vi "Add_Pitot_Vel.vi"(1 "Channels from Client In":string[][](array[string])=[["Data Base:Measurement:Type", "LDA & Cw"], ["Data Base:Position:No of Inst", "2"], ["Data Base:Position:X1", "-60"], ["Data Base:Position:X2", ""], ["Data Base:Position:Y1", "2"], ["Data Base:Position:Y2", "0.00"], ["Data Base:Position:Z1", "0.00"], ["Data Base:Position:Z2", "2.00"]]) -> (0 "Channels from Client Out":string[][](array[string])=[["Data Base:Measurement:Type", "LDA & Cw"], ["Data Base:Position:No of Inst", "2"], ["Data Base:Position:X1", "-60"], ["Data Base:Position:X2", ""], ["Data Base:Position:Y1", "2"], ["Data Base:Position:Y2", "0.00"], ["Data Base:Position:Z1", "0.00"], ["Data Base:Position:Z2", "2.00"]])   [LabVIEW 2011]
uses:
  ADAM Client/Sub VIs/ADAM Controls/Update_scan_value.ctl
  Globals/Meas_global.vi
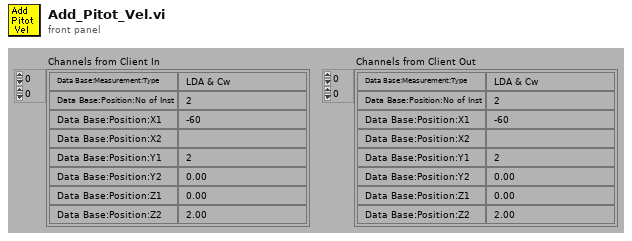
[diagram p1: front panel]
types:
  T1 = typedef "Update_scan_value.ctl" = cluster{"Channel Name":string, "New Value":dbl}
  T2 = typedef "Velocity_cluster.ctl" = cluster{"Name":string, "U":dbl, "u^2":dbl, "u^3/(u^2)^(1.5)":dbl, "u^4/(u^2)^2 -3":dbl, "% u'/U":dbl, "Mean % Err":dbl, "u^4":dbl}
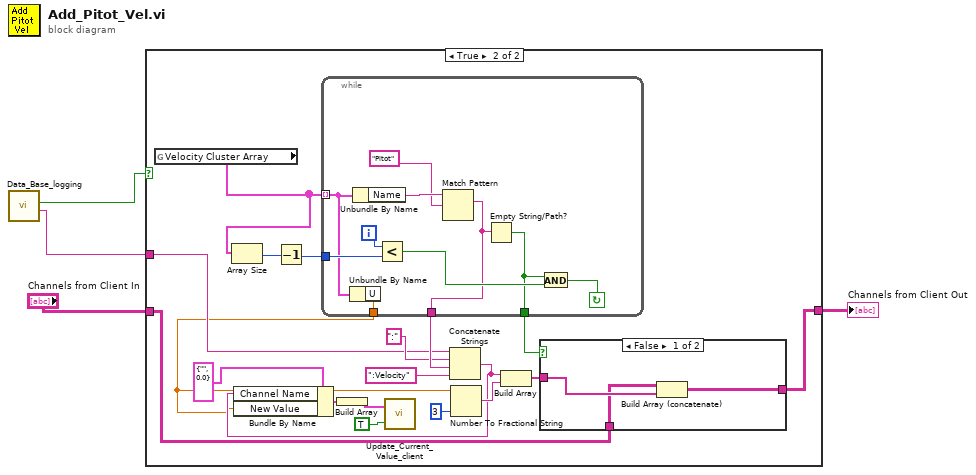
[diagram p0: block diagram]
diagram:
  n1 = call "Data_Base_logging.vi"() -> ("Close Loop with Pitot?"=w2:bool, "Rig Name"=w1:string)  [unwired: 3 out]
  n2 = case shown="True" w2 {
    tunnel: "Channels from Client In" -> [w5 w14]
    tunnel: [w5 w13] -> w3
    tunnel: w1 -> [_ w12]
    frame False {
    }
    frame True {
      n3 = global read "Meas_global.vi" "Velocity Cluster Array"() -> (w24:T2[])
      n4 = Array Size(array=w24) -> (size(s)=w23:i32)
      n5 = Decrement(x=w23) -> (x-1=w22:i32)
      n6 = while {
        tunnel: [w25] -> w8
        tunnel: [w26] -> w20
        tunnel: [w28] -> w21
        tunnel: w22 -> [w33]
        tunnel: w24 -> [w29] mode=indexing
        i -> [w34]
        stop <- w30 continue-if-true
        n7 = Unbundle By Name(w29) -> ("U"=w25:dbl)
        n8 = Unbundle By Name(w29) -> ("Name"=w32:string)
        n9 = Less?(x=w34, y=w33) -> (x < y?=w31:bool)
        n10 = Match Pattern(string=w32, regular expression="Pitot") -> (match substring=w26:string)  [unwired: 4 out]
        n11 = Empty String/Path?(string/path=w26) -> (empty?=w28:bool)
        n12 = And(x=w28, y=w31) -> (x .and. y?=w30:bool)
      }
      n13 = Concatenate Strings(w12, ":" ("Substring"), w20, ":Velocity" ("Substring")) -> (w9:string)
      n14 = Bundle By Name(cluster=T1 {"Channel Name"="", "New Value"=0.0} ("Update Scan Value Cluster"), "Channel Name"=w9, "New Value"=w8) -> (w7:T1)
      n15 = Build Array(w7) -> (w6:T1[])
      n16 = call "Update_Current_Value_client.vi"("Don't Bother with check?"=TRUE, "Update array in"=w6) -> ()
      n17 = Number To Fractional String(number=w8, precision (6)=i16 3) -> (F-format string=w16:string)  [unwired: 2 out]
      n18 = Build Array(w9, w16) -> (w15:string[])
      n19 = case shown="False" w21 {
        tunnel: w15 -> [w37 _]
        tunnel: w14 -> [w36 w38]
        tunnel: [w35 w38] -> w13
        frame False {
          n20 = Build Array (concatenate)(w36, w37) -> (w35:string[][])
        }
        frame True {
        }
      }
    }
  }
  "Channels from Client Out" <- w3
